vi "readPress01.vi"() -> ()   [LabVIEW 2011]
uses:
  Growth Sequences/Control 1.ctl
panel:
  out "reference out":T1="COM1"
  in  "delay before read (ms)":u32=500
  in  "y":i32=1000
  in  "VISA resource name":T1="COM1"
  out "read buffer":string
  out "P (Torr)":dbl
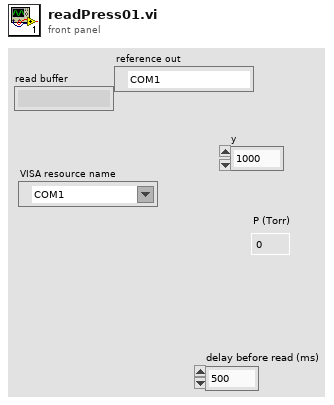
[diagram p1: front panel]
types:
  T1 = typedef "Control 1.ctl" = refnum<visa-resource-name>
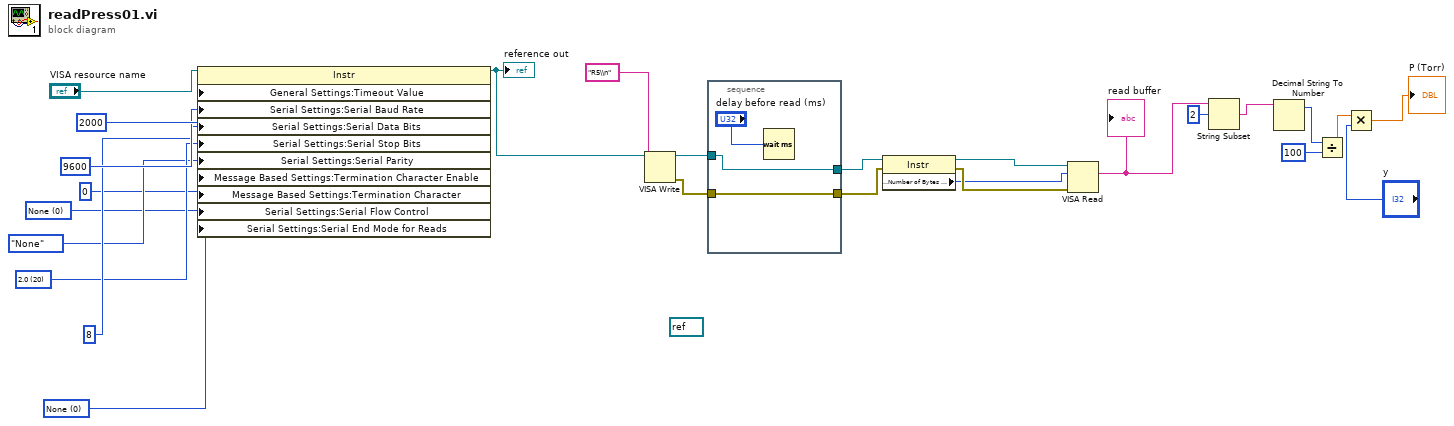
[diagram p0: block diagram]
diagram:
  w2 = u16 0 items=["None", "Last Bit", "TermChar"] ("Serial Settings:End Mode for Reads")
  w3 = u16 0 items=["None", "XON/XOFF", "RTS/CTS", "XON/XOFF & RTS/CTS", "DTR/DSR", "XON/XOFF & DTR/DSR"] ("Serial Settings:Flow Control")
  (unwired) refnum<visa-resource-name> refnum ("VISA resource name out")
  w6 = u16 20 items=["1.0"=10, "1.5"=15, "2.0"=20] ("stop bits (10: 1 bit)")
  n1 = property class="Instr" props=["General Settings:Timeout Value", "Serial Settings:Serial Baud Rate", "Serial Settings:Serial Data Bits", "Serial Settings:Serial Stop Bits", "Serial Settings:Serial Parity", "Message Based Settings:Termination Character Enable", "Message Based Settings:Termination Character", "Serial Settings:Serial Flow Control", "Serial Settings:Serial End Mode for Reads"](reference="VISA resource name", "General Settings:Timeout Value"=u32 2000, "Serial Settings:Serial Baud Rate"=u32 9600 ("baud rate (9600)"), "Serial Settings:Serial Data Bits"=u16 8 ("data bits (8)"), "Serial Settings:Serial Stop Bits"=w6, "Serial Settings:Serial Parity"=enum16{"None", "Odd", "Even", "Mark", "Space"}."None" ("parity (0:none)"), "Message Based Settings:Termination Character"=u8 0, "Serial Settings:Serial Flow Control"=w3, "Serial Settings:Serial End Mode for Reads"=w2) -> (reference out=w1:T1)  [unwired: 2 in, 1 out]
  "reference out" <- w1
  n2 = VISA Write(VISA resource name=w1, write buffer="R5\\n") -> (VISA resource name out=w17:T1, error out=w16:errorcluster)  [unwired: 1 in, 1 out]
  n3 = stacked-sequence {
    tunnel: w16 -> [w29]
    tunnel: [w29] -> w14
    tunnel: [w27] -> w15
    tunnel: w17 -> [w27]
    frame #0 {
      n4 = Wait (ms)(milliseconds to wait="delay before read (ms)") -> ()  [unwired: 1 out]
    }
  }
  n5 = property class="Instr"(reference=w15, error in=w14) -> (reference out=w12:T1, error out=w13:errorcluster, "Serial Settings:Number of Bytes at Serial Port"=w11:u32)
  n6 = VISA Read(VISA resource name=w12, byte count=w11, error in (no error)=w13) -> (read buffer=w26:string)  [unwired: 3 out]
  "read buffer" <- w26
  n7 = String Subset(string=w26, offset (0)=2) -> (substring=w25:string)  [unwired: 1 in]
  n8 = Decimal String To Number(string=w25) -> (offset past number=w20:i32)  [unwired: 2 in, 1 out]
  n9 = Divide(x=w20, y=100) -> (x/y=w18:dbl)
  n10 = Multiply(x=w18, y="y") -> (x*y=→"P (Torr)":dbl)
